vi "Initiate Updates.vi"(8 "error in (no error)":errorcluster, 11 "IViewable In":refnum<class "IViewable.lvclass">) -> (0 "error out":errorcluster, 3 "IViewable Out":refnum<class "IViewable.lvclass">)   [LabVIEW 2015, in "IViewable.lvlib" / "IViewable.lvclass"]
uses:
  IViewable.lvclass
  IViewable.lvclass/IViewable.ctl
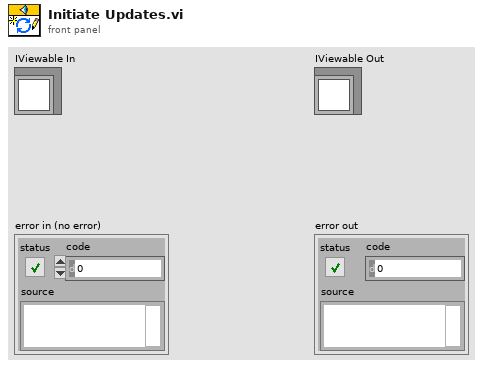
[diagram p1: front panel]
types:
  T1 = enum32{"Invalid", "Standard", "Closed", "Hidden", "Minimized", "Maximized"}
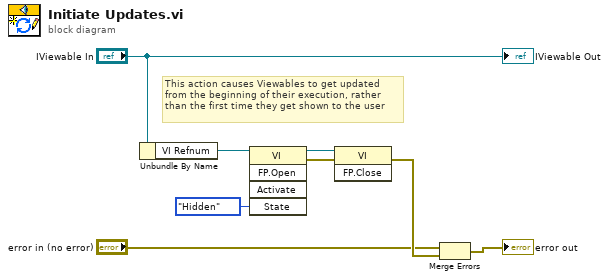
[diagram p0: block diagram]
diagram:
  # "This action causes Viewables to get updated\nfrom the beginning of their execution, rather\nthan the first time they get shown to the user"
  n1 = Unbundle By Name("IViewable In") -> ("VI Refnum"=w3:refnum<vi>)
  n2 = invoke class="VI" method="FP.Open"(reference=w3, "State"=T1."Hidden") -> (reference out=w5:refnum<vi>, error out=w6:errorcluster)  [unwired: 3 in, 3 out]
  n3 = invoke class="VI" method="FP.Close"(reference=w5, error in=w6) -> (error out=w8:errorcluster)  [unwired: 1 in, 2 out]
  n4 = Merge Errors("error in (no error)", w8) -> (→"error out":errorcluster)
  "IViewable Out" <- "IViewable In"
